vi "Leftovers remove.vi"(7 "Leftovers":T2(array[cluster]), 10 "Secondary hits in":T2(array[cluster]), 11 "Primary hits in":T1) -> (2 "Secondary hits out":T2(array[cluster]), 3 "Primary hits out":T1, 5 "Primary ID":i8)   [LabVIEW 2016]
uses:
  Global Variables/System info.vi
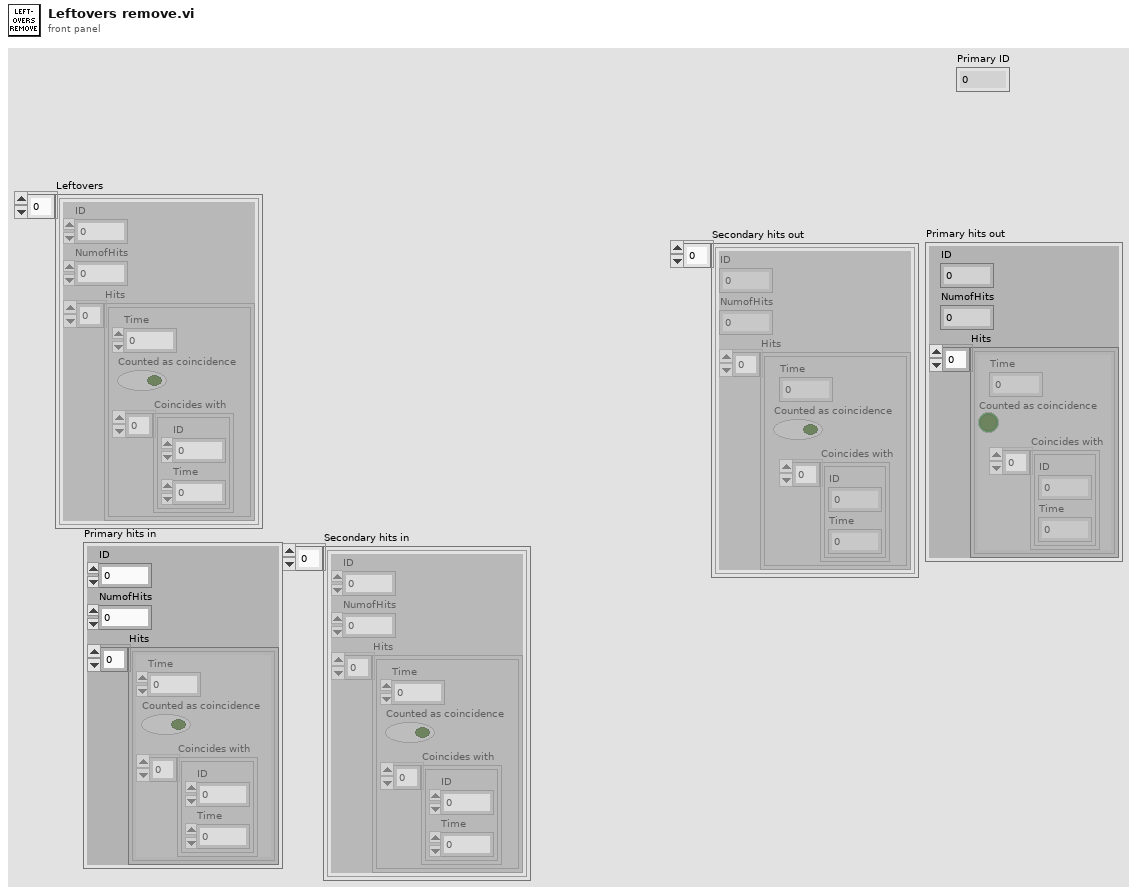
[diagram p1: front panel]
types:
  T1 = cluster{"ID":i8, "NumofHits":i32, "Hits":cluster{"Time":u64, "Counted as coincidence":bool, "Coincides with":cluster{"ID":i8, "Time":u64}[]}[]}
  T2 = cluster{"ID":i8, "NumofHits":i32, "Hits":cluster{"Time":u64, "Counted as coincidence":bool, "Coincides with":cluster{"ID":i8, "Time":u64}[]}[]}[]
  T3 = cluster{"Time":u64, "Counted as coincidence":bool, "Coincides with":cluster{"ID":i8, "Time":u64}[]}[]
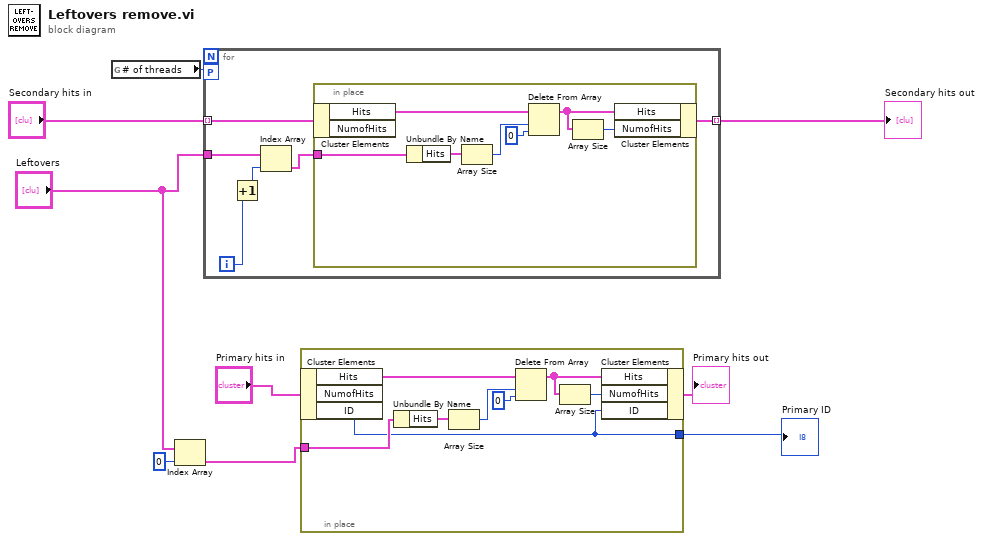
[diagram p0: block diagram]
diagram:
  n1 = global read "System info.vi" "# of threads"() -> (w7:i32)
  n2 = Index Array(array="Leftovers", index=0) -> (element=w3:T1)
  n3 = for {
    tunnel: "Secondary hits in" -> [w15] mode=indexing
    tunnel: [w14] -> w9 mode=indexing
    tunnel: "Leftovers" -> [w13]
    workers-P: w7 -> [_]
    i -> [w11]
    n4 = Increment(x=w11) -> (x+1=w10:i32)
    n5 = Index Array(array=w13, index=w10) -> (element=w12:T1)
    n6 = in-place {
      in-place-border: w12 -> [w16]
      n7 = in-place-cluster #1(w15) -> ("Hits"=w22:T3)  [unwired: 1 out]
      n8 = Unbundle By Name(w16) -> ("Hits"=w21:T3)
      n9 = Array Size(array=w21) -> (size(s)=w20:i32)
      n10 = Delete From Array(array=w22, length=w20, index=0) -> (array with subset deleted=w17:T3)  [unwired: 1 out]
      n11 = Array Size(array=w17) -> (size(s)=w18:i32)
      n12 = in-place-cluster #1("Hits"=w17, "NumofHits"=w18) -> (w14:T1)
    }
  }
  "Secondary hits out" <- w9
  n13 = in-place {
    in-place-border: w3 -> [w24]
    in-place-border: [w23] -> w1
    n14 = in-place-cluster #2("Primary hits in") -> ("Hits"=w30:T3, "ID"=w23:i8)  [unwired: 1 out]
    n15 = Unbundle By Name(w24) -> ("Hits"=w29:T3)
    n16 = Array Size(array=w29) -> (size(s)=w28:i32)
    n17 = Delete From Array(array=w30, length=w28, index=0) -> (array with subset deleted=w25:T3)  [unwired: 1 out]
    n18 = Array Size(array=w25) -> (size(s)=w26:i32)
    n19 = in-place-cluster #2("Hits"=w25, "NumofHits"=w26, "ID"=w23) -> (→"Primary hits out":T1)
  }
  "Primary ID" <- w1
